vi "LabVIEWModbusRTU.vi"() -> ()   [LabVIEW 2019]
uses:
  <vilib>/Modbus/master/Create Master Instance (Serial).vi
  <vilib>/Modbus/master/Modbus Master.lvclass
panel:
  out "Temperature":u16 caption="register"
  in  "Relais":u16
  in  "Bouton Stop":bool
  in  "unit ID":u8=1
  in  "VISA resource name":refnum<visa-resource-name>
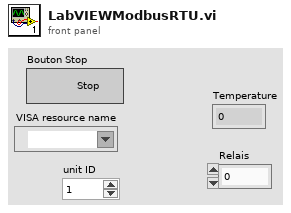
[diagram p1: front panel]
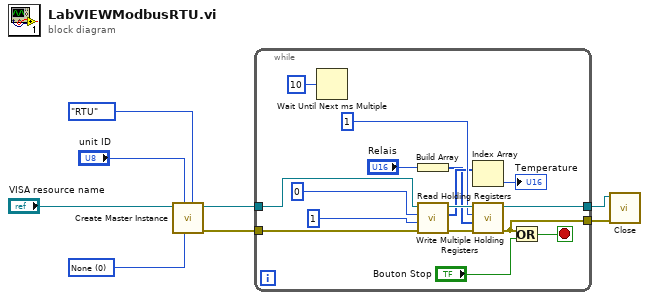
[diagram p0: block diagram]
diagram:
  w6 = u16 0 items=["None", "Odd", "Even"] ("parity (Even)")
  n1 = call-poly <vilib>:"Create Master Instance.vi"("serial type"=enum16{"RTU", "ASCII"}."RTU", "parity (Even)"=w6, "unit ID"="unit ID", "VISA resource name"="VISA resource name") -> ("error out"=w1:errorcluster, "serial master instance"=w4:refnum<class "Modbus Master.lvclass">)  [unwired: 6 in]
  n2 = while {
    tunnel: w4 -> [w24]
    tunnel: [w10] -> w3
    tunnel: [w14] -> w2
    tunnel: w1 -> [w12]
    stop <- w11 stop-if-true
    n3 = Wait Until Next ms Multiple(millisecond multiple=u32 10 ("n millisecondes")) -> ()  [unwired: 1 out]
    n4 = Build Array("Relais") -> (w15:u16[])
    n5 = call-dynamic "Read Holding Registers.vi"("error in (no error)"=w12, "number of holding registers"=u16 1, "starting address"=u16 0, "Modbus master in"=w24) -> ("error out"=w20:errorcluster, "register values"=w18:u16[], "Modbus master out"=w21:refnum<class "Modbus Master.lvclass">)  [unwired: 5 in]
    n6 = Index Array(array=w18) -> (element=→"Temperature":u16)  [unwired: 1 in]
    n7 = call-dynamic "Write Multiple Holding Registers.vi"("error in (no error)"=w20, "holding register values"=w15, "starting address"=u16 1, "Modbus master in"=w21) -> ("error out"=w10:errorcluster, "Modbus master out"=w14:refnum<class "Modbus Master.lvclass">)  [unwired: 6 in]
    n8 = Or(x=w10, y="Bouton Stop") -> (x .or. y?=w11:bool)
  }
  n9 = call-dynamic "Close.vi"("error in (no error)"=w3, "Modbus master in"=w2) -> ()  [unwired: 9 in, 1 out]
